vi "open MB.vi"(4 "Port (502)":u16=502, 6 "IP Address":string="localhost", 7 "MODE":u16(ring) items=["Modbus RTU", "Modbus TCP"], 8 "error in (no error)":errorcluster caption="错误输入（无错误）", 9 "Serial Config":T1={"baud rate (bps)"=19200, "stop bits"=10, "parity"=0, "flow control"=0, "timeout"=1000, "retries"=1} {"stop bits" items=["1.0"=10, "1.5"=15, "2.0"=20]; "parity" items=["None", "Odd", "Even", "Mark", "Space"]; "flow control" items=["None", "XON/XOFF", "RTS/CTS", "XON/XOFF & RTS/CTS", "DTR/DSR", "XON/XOFF & DTR/DSR"]}, 10 "Slave ID":u8=1, 11 "VISA资源名称":refnum<visa-resource-name>) -> (0 "error out":errorcluster caption="错误输出", 3 "MB session out":refnum<class "MB_Master.lvclass">)   [LabVIEW 2022 SP3, in "斯坦道多参数.lvlib"]
uses:
  <vilib>/Plasmionique/MB Master/MB_Master/MB_Master.lvclass
  <vilib>/Plasmionique/MB Master/MB_Master_Serial/MB_Master_Serial.lvclass
  C:/Program Files (x86)/National Instruments/LabVIEW 2022/vi.lib/Plasmionique/MB Master/MB_Master/MB_Master.lvclass
  <vilib>/Plasmionique/MB Master/MB_Master_TCP/MB_Master_TCP.lvclass
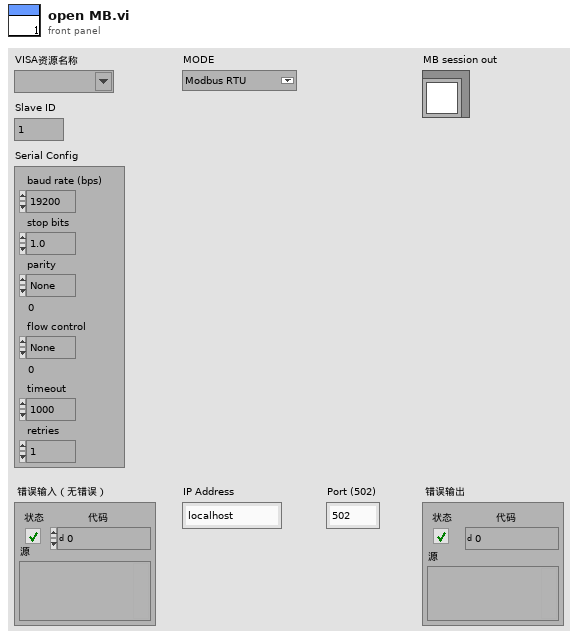
[diagram p1: front panel]
types:
  T1 = cluster{"baud rate (bps)":u32, "stop bits":u16, "parity":u16, "flow control":u16, "timeout":u32, "retries":i32}
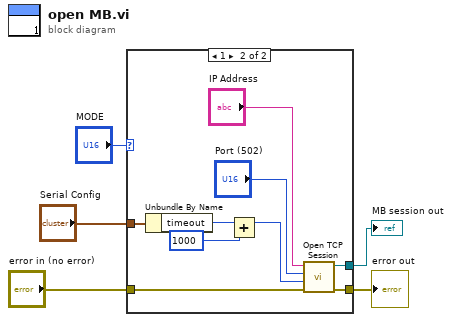
[diagram p0: block diagram]
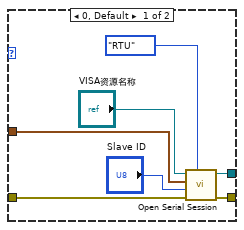
[diagram p2: hidden frame]
diagram:
  n1 = case shown="1" "MODE" {
    tunnel: "error in (no error)" -> [w9 w21]
    tunnel: [w8 w20] -> w4
    tunnel: [w7 w19] -> w2
    tunnel: "Serial Config" -> [w6 w16]
    frame 0, Default {
      n2 = call <vilib>:"Open Serial Session.vi"("Mode (RTU)"=enum16{"RTU", "ASCII"}."RTU", "Error in"=w9, "Slave ID"="Slave ID", "Serial Config"=w6, "VISA Resource"="VISA资源名称") -> ("Error out"=w8:errorcluster, "MB_Serial session"=w7:refnum<class "MB_Master_Serial.lvclass">)  [unwired: 5 in]
    }
    frame 1 {
      n3 = Unbundle By Name(w16) -> ("timeout"=w15:u32)
      n4 = Add(x=w15, y=u32 1000) -> (x+y=w14:u32)
      n5 = call <vilib>:"Open TCP Session.vi"("error in (no error)"=w21, "Timeout (10000)"=w14, "Port (502)"="Port (502)", "IP Address"="IP Address") -> ("error out"=w20:errorcluster, "MB_TCP session"=w19:refnum<class "MB_Master_TCP.lvclass">)  [unwired: 6 in]
    }
  }
  "error out" <- w4
  "MB session out" <- w2
